vi "PicoErrorString.vi"(4 "error in":errorcluster) -> (0 "[user-defined descriptions]":string[](array[string]), 1 "String":string, 3 "[user-defined codes]":u32[](array[numeric])=[5001, 5002, 5003, 5004, 5005, 5006, 5007, 5008, 5009, 5010, 5011, 5012, 5013, 5014, 5015, 5016, 5017, 5018, 5019, 5020, 5021, 5022, 5023, 5024, 5025, 5026, 5027, 5028, 5029, 5030, 5031, 5032, 5033, 5034, 5035, 5036, 5037, 5038, 5039, 5040, 5041, 5042, 5043, 5044, 5045, 5046, 5047, 5048, 5049, 5050, 5051, 5052, 5053, 5054, 5055, 5056, 5057, 5058, 5059, 5060, 5061, 5063, 5064, 5065, 5066, 5067, 5068, 5069, 5070, 5071, 5072, 5073, 5074, 5075, 5076, 5077, 5078, 5079, 5080, 5081, 5082, 5083, 5084, 5086, 5087, 5088, 5089, 5259, 5260, 5261, 5262, 5263, 5264, 5265, 5266, 5267, 5268, 5269, 5270, 5271, 5272, 5273, 5274, 5275, 5276, 5277, 5278, 5279, 5280, 5281, 5282, 5283, 5284, 5285, 5286, 5287, 5288, 5289, 5290, 5291, 5292, 5293, 5294, 5295, 5296, 5297, 5298, 5299, 5300, 5301, 5302, 5303, 5304, 5305, 5306, 5307, 5308, 5309, 5310, 5311, 5312, 5313, 5314, 5315, 5316, 5317, 5318, 5319, 5320, 5321, 5090, 5091, 5092, 5093, 5094, 5095, 5096, 5097, 5322, 5323, 5324, 5325, 5326, 5327, 5328, 5329, 5330, 5331, 5332, 5333, 5334, 5335, 5336, 5337, 5338, 5339, 5340, 5341, 5342, 5343, 16782216, 268440456, 268440457, 268440458, 268440459, 268440460, 268440461, 268440462, 268440463, 268440464, 285217672])   [LabVIEW 2020]
doc: "This VI takes an error cluster and if an error has occurred, displays a message box indicating the source of the error and the status code returned by the driver."
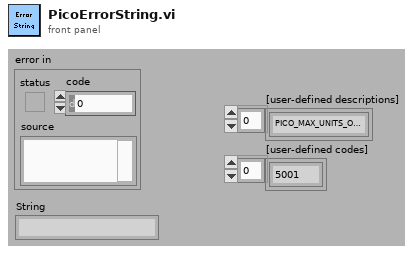
[diagram p1: front panel]
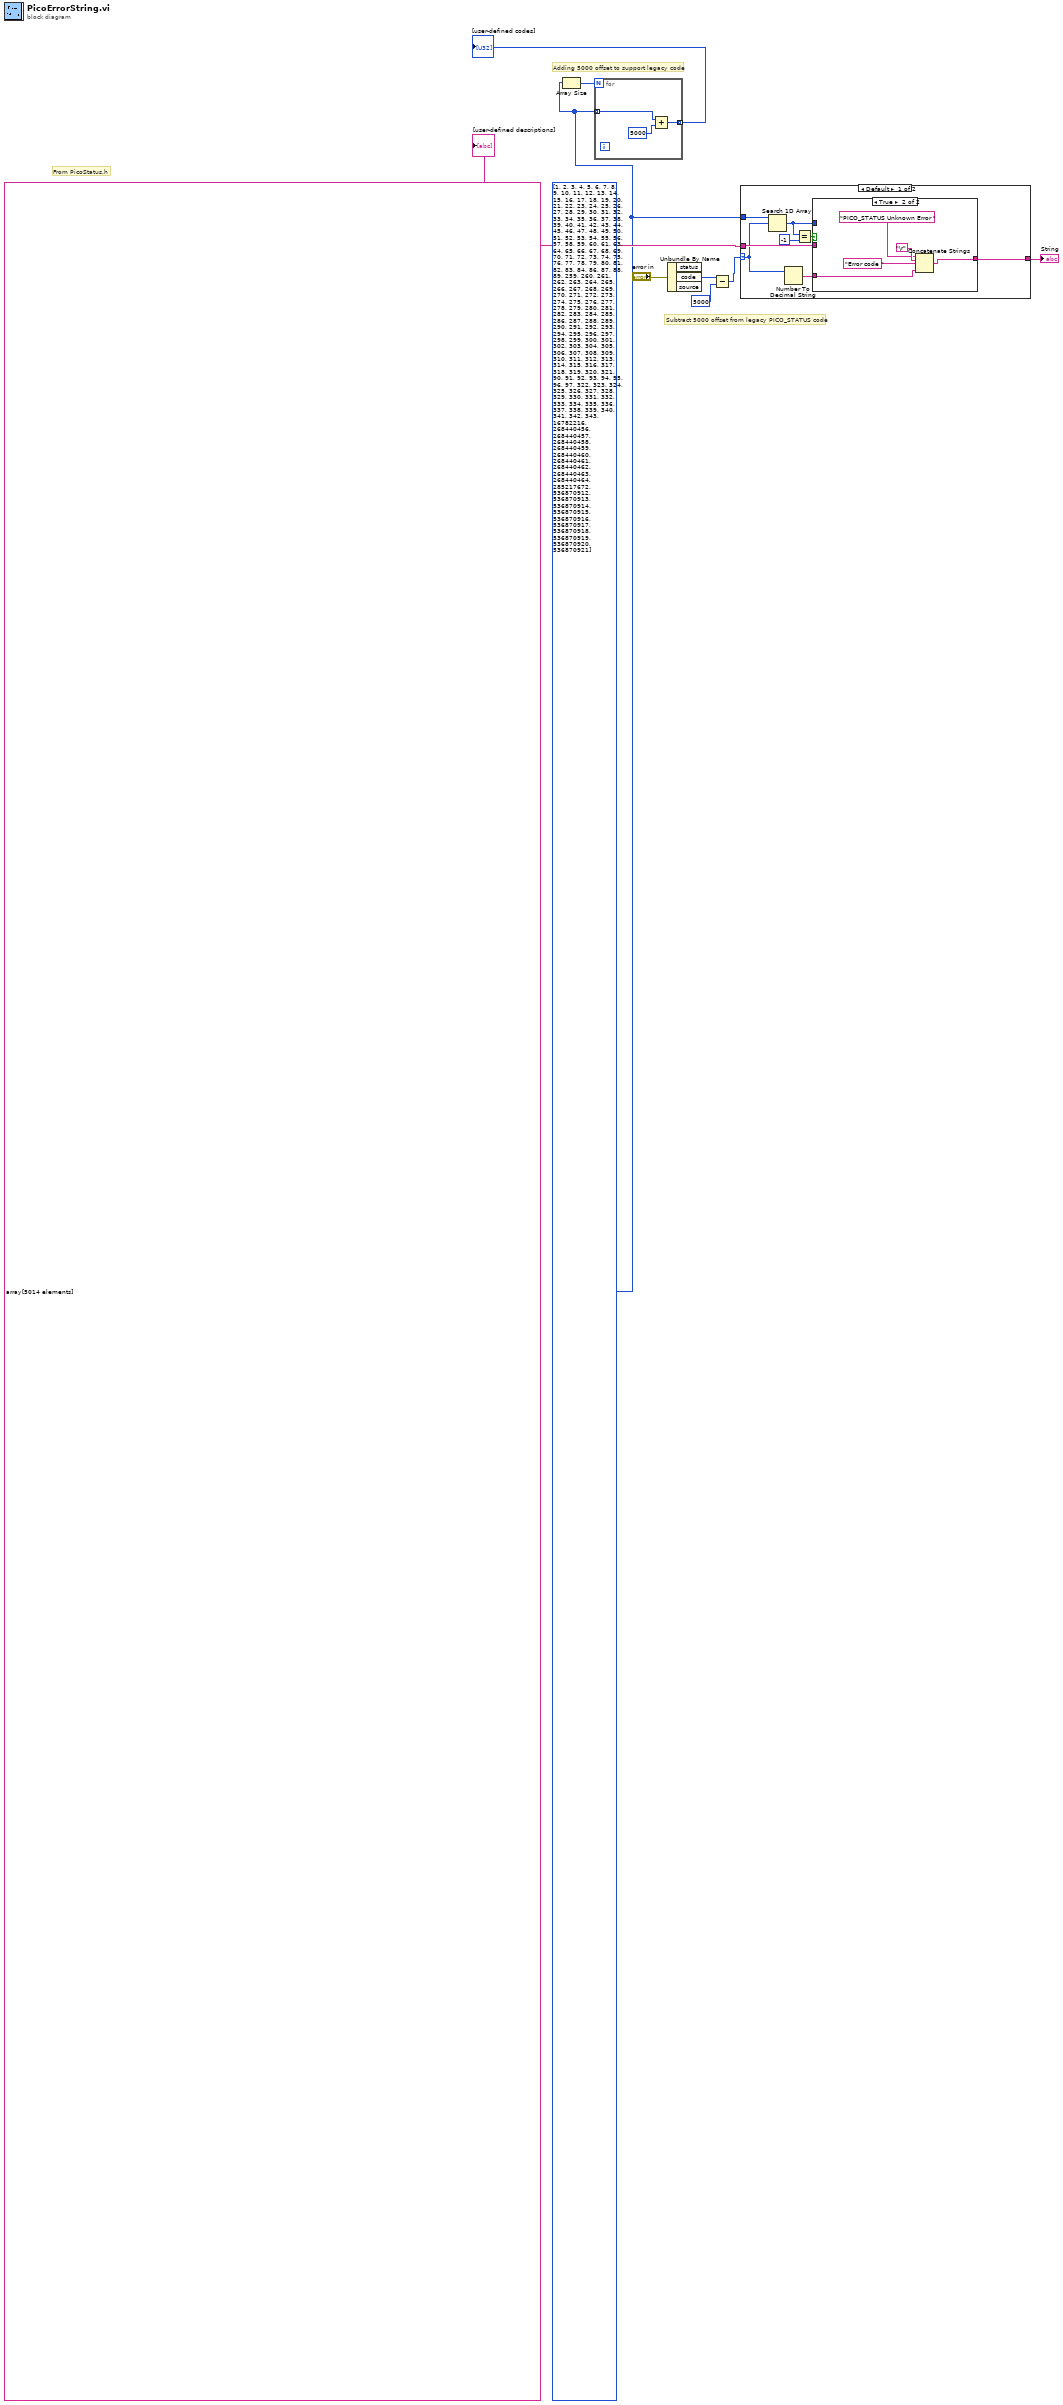
[diagram p0: block diagram]
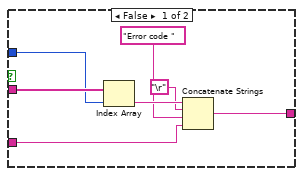
[diagram p2: hidden frame]
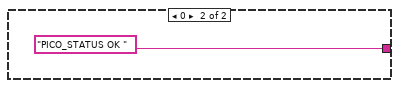
[diagram p3: hidden frame]
diagram:
  w4 = u32[] [1, 2, 3, 4, 5, 6, 7, 8, 9, 10, 11, 12, 13, 14, 15, 16, 17, 18, 19, 20, 21, 22, 23, 24, 25, 26, 27, 28, 29, 30, 31, 32, 33, 34, 35, 36, 37, 38, 39, 40, 41, 42, 43, 44, 45, 46, 47, 48, 49, 50, 51, 52, 53, 54, 55, 56, 57, 58, 59, 60, 61, 63, 64, 65, 66, 67, 68, 69, 70, 71, 72, 73, 74, 75, 76, 77, 78, 79, 80, 81, 82, 83, 84, 86, 87, 88, 89, 259, 260, 261, 262, 263, 264, 265, 266, 267, 268, 269, 270, 271, 272, 273, 274, 275, 276, 277, 278, 279, 280, 281, 282, 283, 284, 285, 286, 287, 288, 289, 290, 291, 292, 293, 294, 295, 296, 297, 298, 299, 300, 301, 302, 303, 304, 305, 306, 307, 308, 309, 310, 311, 312, 313, 314, 315, 316, 317, 318, 319, 320, 321, 90, 91, 92, 93, 94, 95, 96, 97, 322, 323, 324, 325, 326, 327, 328, 329, 330, 331, 332, 333, 334, 335, 336, 337, 338, 339, 340, 341, 342, 343, 16782216, 268440456, 268440457, 268440458, 268440459, 268440460, 268440461, 268440462, 268440463, 268440464, 285217672, 536870912, 536870913, 536870914, 536870915, 536870916, 536870917, 536870918, 536870919, 536870920, 536870921] ("[user-defined codes]")
  w7 = string[] array[5014 elements] ("[user-defined descriptions]")
  # "Subtract 5000 offset from legacy PICO_STATUS code"
  # "Adding 5000 offset to support legacy code"
  # "From PicoStatus.h"
  n1 = Array Size(array=w4) -> (size(s)=w6:i32)
  n2 = for {
    N: w6 -> [_]
    tunnel: w4 -> [w10] mode=indexing
    tunnel: [w11] -> w5 mode=indexing
    n3 = Add(x=w10, y=u32 5000) -> (x+y=w11:u32)
  }
  "[user-defined codes]" <- w5
  n4 = Unbundle By Name("error in") -> ("code"=w3:i32)  [unwired: 2 out]
  n5 = Subtract(x=w3, y=5000) -> (x-y=w2:i32)
  n6 = case shown="Default" w2 {
    selector: w2 -> [w17 _]
    tunnel: w7 -> [w20 _]
    tunnel: w4 -> [w19 _]
    tunnel: [w18 "PICO_STATUS OK " ("string")] -> w8
    frame Default {
      n7 = Search 1D Array(1D array=w19, element=w17) -> (index of element=w15:i32)  [unwired: 1 in]
      n8 = Number To Decimal String(number=w17) -> (decimal integer string=w13:string)  [unwired: 1 in]
      n9 = Equal?(x=w15, y=-1) -> (x = y?=w16:bool)
      n10 = case shown="True" w16 {
        tunnel: w20 -> [w27 _]
        tunnel: w15 -> [w26 _]
        tunnel: [w24 w31] -> w18
        tunnel: w13 -> [w21 w28]
        frame False {
          n11 = Index Array(array=w27, index=w26) -> (element=w25:string)
          n12 = Concatenate Strings(w25, "\r", "Error code " ("string"), w21) -> (w24:string)
        }
        frame True {
          n13 = Concatenate Strings("PICO_STATUS Unknown Error " ("string"), "\r", "Error code " ("string"), w28) -> (w31:string)
        }
      }
    }
    frame 0 {
    }
  }
  "String" <- w8
  "[user-defined descriptions]" <- w7
